vi "CAN MESSAGE WITHOUT START SESSION.vi"(0 "Write":refnum<k21>, 1 "Read":refnum<k21>, 2 "CAN frame":T1 {"payload" format="%x"; "timestamp" format="%<%.7X\n%x>T"; "type" items=["CAN Data"=0, "CAN Remote"=1, "CAN Bus Error"=2, "CAN 2.0 Data"=8, "CAN FD Data"=16, "CAN FD+BRS Data"=24, "J1939 Data"=192, "Delay"=224, "Log Trigger"=225, "Start Trigger"=226]; "identifier" format="%x"}) -> (3 "cluster":T3 {"data[0]"."payload" format="%x"; "data[0]"."timestamp" format="%<%.7X\n%x>T"; "data[0]"."type" items=["CAN Data"=0, "CAN Remote"=1, "CAN Bus Error"=2, "CAN 2.0 Data"=8, "CAN FD Data"=16, "CAN FD+BRS Data"=24, "J1939 Data"=192, "Delay"=224, "Log Trigger"=225, "Start Trigger"=226]; "data[0]"."identifier" format="%x"; "data[1]"."payload" format="%x"; "data[1]"."timestamp" format="%<%.7X\n%x>T"; "data[1]"."type" items=["CAN Data"=0, "CAN Remote"=1, "CAN Bus Error"=2, "CAN 2.0 Data"=8, "CAN FD Data"=16, "CAN FD+BRS Data"=24, "J1939 Data"=192, "Delay"=224, "Log Trigger"=225, "Start Trigger"=226]; "data[1]"."identifier" format="%x"; "data[2]"."payload" format="%x"; "data[2]"."timestamp" format="%<%.7X\n%x>T"; "data[2]"."type" items=["CAN Data"=0, "CAN Remote"=1, "CAN Bus Error"=2, "CAN 2.0 Data"=8, "CAN FD Data"=16, "CAN FD+BRS Data"=24, "J1939 Data"=192, "Delay"=224, "Log Trigger"=225, "Start Trigger"=226]; "data[2]"."identifier" format="%x"; "data[3]"."payload" format="%x"; "data[3]"."timestamp" format="%<%.7X\n%x>T"; "data[3]"."type" items=["CAN Data"=0, "CAN Remote"=1, "CAN Bus Error"=2, "CAN 2.0 Data"=8, "CAN FD Data"=16, "CAN FD+BRS Data"=24, "J1939 Data"=192, "Delay"=224, "Log Trigger"=225, "Start Trigger"=226]; "data[3]"."identifier" format="%x"; "data[4]"."payload" format="%x"; "data[4]"."timestamp" format="%<%.7X\n%x>T"; "data[4]"."type" items=["CAN Data"=0, "CAN Remote"=1, "CAN Bus Error"=2, "CAN 2.0 Data"=8, "CAN FD Data"=16, "CAN FD+BRS Data"=24, "J1939 Data"=192, "Delay"=224, "Log Trigger"=225, "Start Trigger"=226]; "data[4]"."identifier" format="%x"; "data[5]"."payload" format="%x"; "data[5]"."timestamp" format="%<%.7X\n%x>T"; "data[5]"."type" items=["CAN Data"=0, "CAN Remote"=1, "CAN Bus Error"=2, "CAN 2.0 Data"=8, "CAN FD Data"=16, "CAN FD+BRS Data"=24, "J1939 Data"=192, "Delay"=224, "Log Trigger"=225, "Start Trigger"=226]; "data[5]"."identifier" format="%x"; "data[6]"."payload" format="%x"; "data[6]"."timestamp" format="%<%.7X\n%x>T"; "data[6]"."type" items=["CAN Data"=0, "CAN Remote"=1, "CAN Bus Error"=2, "CAN 2.0 Data"=8, "CAN FD Data"=16, "CAN FD+BRS Data"=24, "J1939 Data"=192, "Delay"=224, "Log Trigger"=225, "Start Trigger"=226]; "data[6]"."identifier" format="%x"; "data[7]"."payload" format="%x"; "data[7]"."timestamp" format="%<%.7X\n%x>T"; "data[7]"."type" items=["CAN Data"=0, "CAN Remote"=1, "CAN Bus Error"=2, "CAN 2.0 Data"=8, "CAN FD Data"=16, "CAN FD+BRS Data"=24, "J1939 Data"=192, "Delay"=224, "Log Trigger"=225, "Start Trigger"=226]; "data[7]"."identifier" format="%x"; "data[8]"."payload" format="%x"; "data[8]"."timestamp" format="%<%.7X\n%x>T"; "data[8]"."type" items=["CAN Data"=0, "CAN Remote"=1, "CAN Bus Error"=2, "CAN 2.0 Data"=8, "CAN FD Data"=16, "CAN FD+BRS Data"=24, "J1939 Data"=192, "Delay"=224, "Log Trigger"=225, "Start Trigger"=226]; "data[8]"."identifier" format="%x"}, 4 "Write":refnum<k21>, 5 "Read":refnum<k21>, 6 "error out":errorcluster)   [LabVIEW 2023]
uses:
  <vilib>/xnet/xnet.llb/XNET Frame CAN.ctl
  <vilib>/xnet/xnet.llb/XNET Frame Type CAN.ctl
  <vilib>/xnet/xnet.llb/XNET Write (Frame CAN).vi
  Sub VIs/Global .vi
  <vilib>/xnet/xnet.llb/XNET Read (Frame CAN).vi
panel:
  out "number":u32 format="%x"
  out "data[0].identifier":u32 format="%x"
  in  "error out 2":errorcluster
  out "data 2":T1[](array[typedef]) {"payload" format="%x"; "timestamp" format="%<%.7X\n%x>T"; "type" items=["CAN Data"=0, "CAN Remote"=1, "CAN Bus Error"=2, "CAN 2.0 Data"=8, "CAN FD Data"=16, "CAN FD+BRS Data"=24, "J1939 Data"=192, "Delay"=224, "Log Trigger"=225, "Start Trigger"=226]; "identifier" format="%x"}
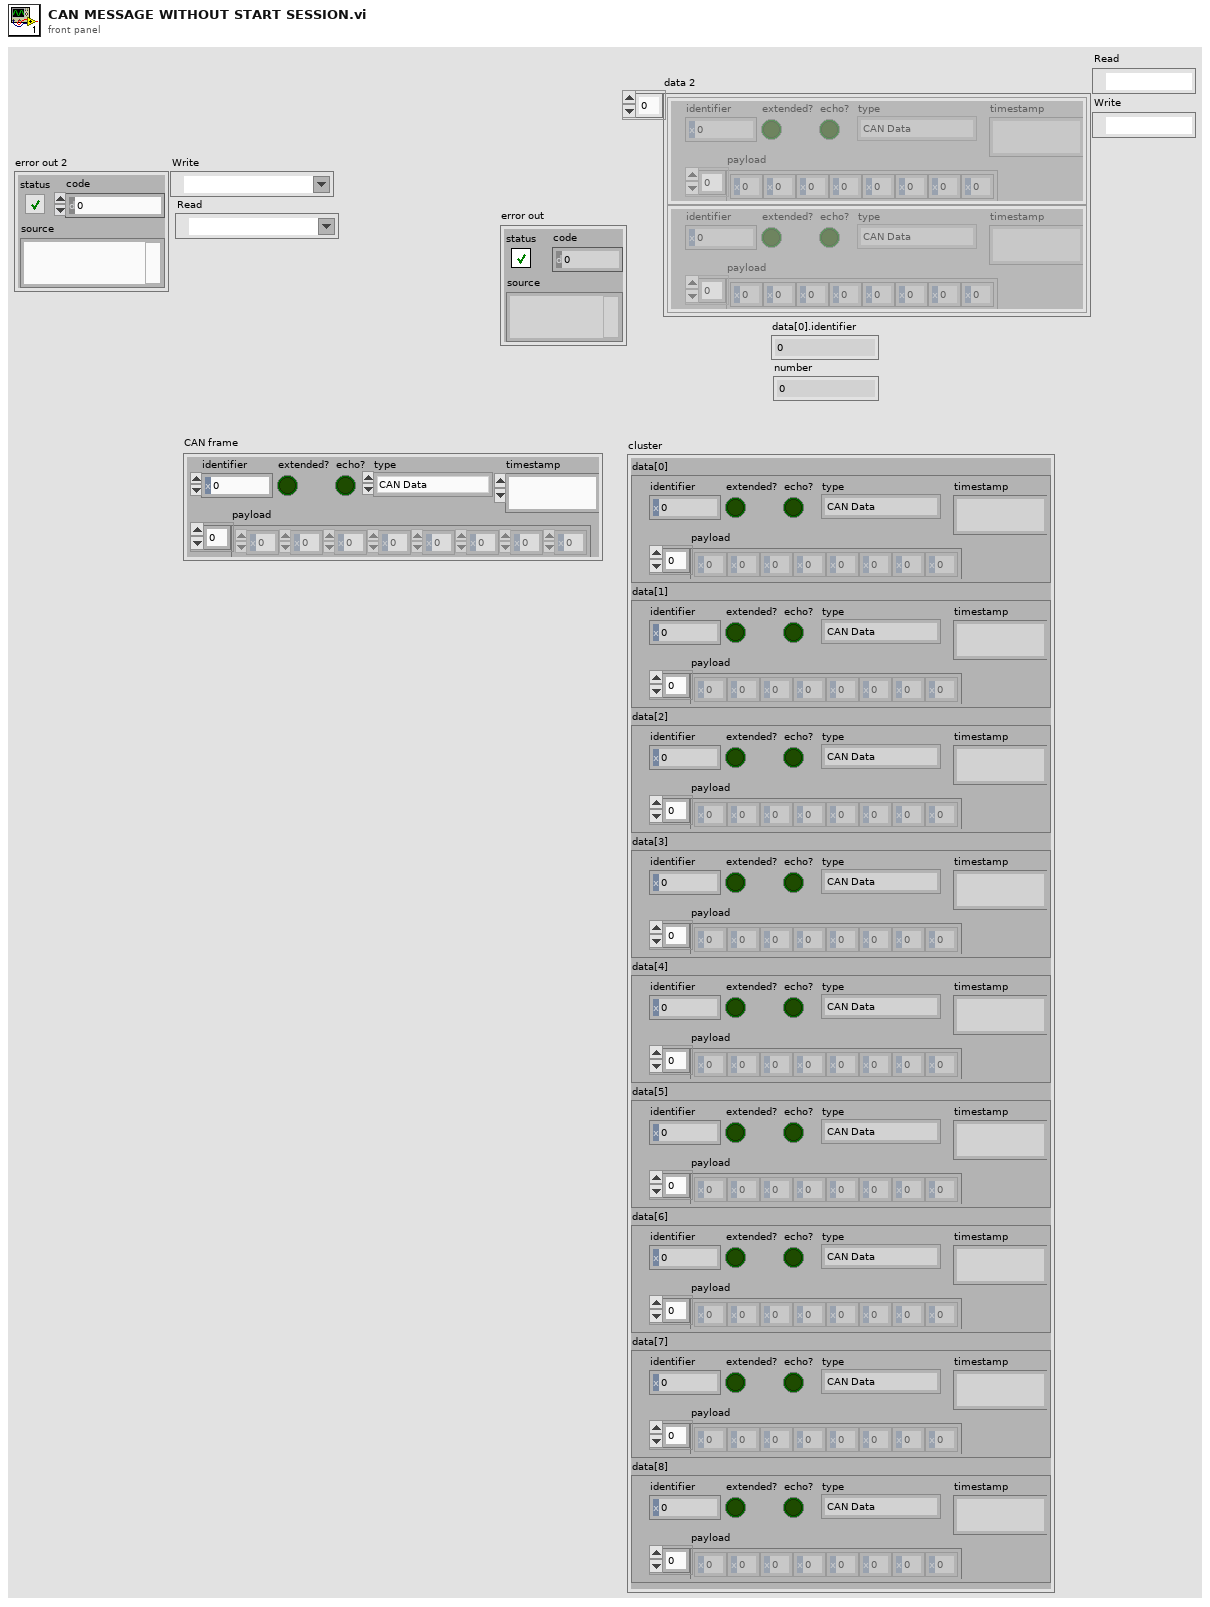
[diagram p1: front panel]
types:
  T1 = typedef "XNET Frame CAN.ctl" = cluster{"timestamp":timestamp, "payload":u8[], "identifier":u32, "type":T2, "extended?":bool, "echo?":bool}
  T2 = typedef "XNET Frame Type CAN.ctl" = u8
  T3 = cluster{"data[0]":T1, "data[1]":T1, "data[2]":T1, "data[3]":T1, "data[4]":T1, "data[5]":T1, "data[6]":T1, "data[7]":T1, "data[8]":T1}
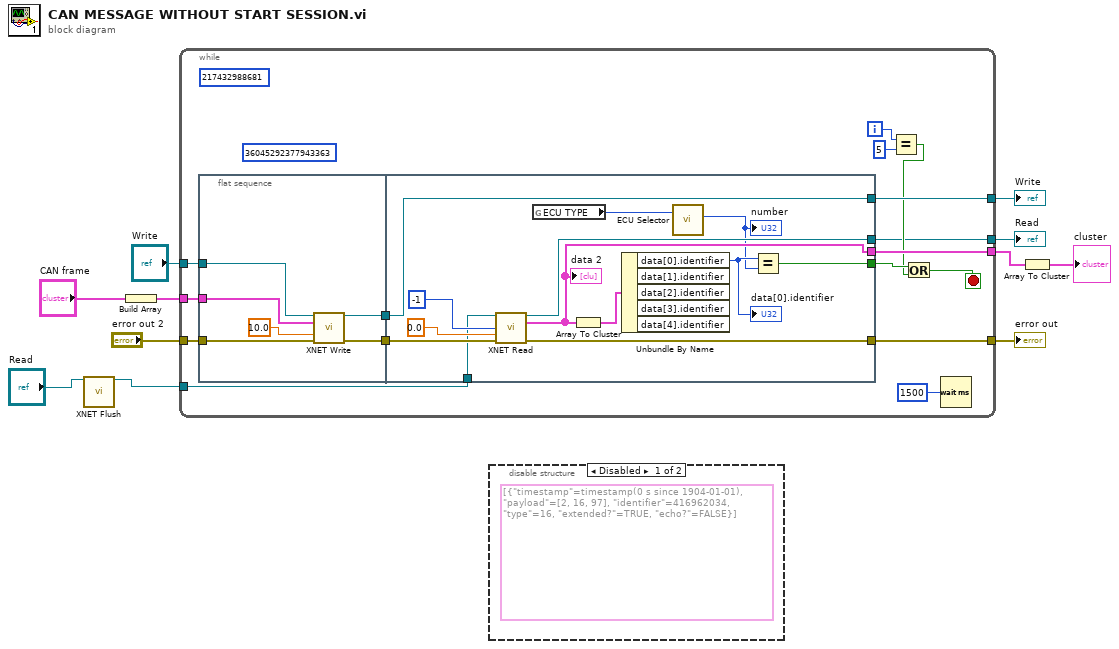
[diagram p0: block diagram]
diagram:
  n1 = call <vilib>:"XNET Flush.vi"("session in"="Read") -> ("session out"=w1:refnum<k21>)  [unwired: 13 in, 1 out]
  n2 = Build Array("CAN frame") -> (w8:T1[])
  n3 = while {
    tunnel: w1 -> [w13]
    tunnel: "Write" -> [w27]
    tunnel: "error out 2" -> [w26]
    tunnel: [w23] -> w7
    tunnel: [w22] -> w11
    tunnel: w8 -> [w21]
    tunnel: [w20] -> w4
    tunnel: [w14] -> w3
    i -> [w17]
    stop <- w12 stop-if-true
    (unwired) u64 36045292377943363 ("Interface:CAN:64bit FD Baud Rate")
    (unwired) u64 217432988681 ("Interface:64bit Baud Rate")
    n4 = flat-sequence {
      tunnel: w27 -> [w33]
      tunnel: w26 -> [w31]
      tunnel: [w30] -> w25
      tunnel: w21 -> [w29]
      tunnel: [w28] -> w19
      tunnel: [w43] -> w18
      tunnel: w25 -> [w42]
      tunnel: w13 -> [w41]
      tunnel: [w40] -> w23
      tunnel: [w39] -> w22
      tunnel: [w37] -> w14
      tunnel: [w36] -> w20
      tunnel: w19 -> [w36]
      frame #0 {
        n5 = call-poly <vilib>:"XNET Write.vi"("session in"=w33, "data"=w29, "timeout (10)"=10.0, "error in (no error)"=w31) -> ("session out"=w28:refnum<k21>, "error out"=w30:errorcluster)  [unwired: 10 in]
      }
      frame #1 {
        n6 = call-poly <vilib>:"XNET Read.vi"("session in"=w41, "number to read (-1)"=-1, "timeout (0)"=0.0, "error in (no error)"=w42) -> ("session out"=w37:refnum<k21>, "data"=w39:T1[], "error out"=w40:errorcluster)  [unwired: 8 in, 1 out]
        "data 2" <- w39
        n7 = global read "Global .vi" "ECU TYPE"() -> (w35:u16)
        n8 = Array To Cluster(array=w39) -> (cluster=w38:T3)
        n9 = Unbundle By Name(w38) -> ("data[0].identifier"=w44:u32)  [unwired: 4 out]
        "data[0].identifier" <- w44
        n10 = call "ECU Selector.vi"("ECU TYPE"=w35) -> ("Numeric Request"=w34:i32)  [unwired: 1 in, 4 out]
        "number" <- w34
        n11 = Equal?(x=w44, y=w34) -> (x = y?=w43:bool)
      }
    }
    n12 = Equal?(x=w17, y=5) -> (x = y?=w16:bool)
    n13 = Or(x=w18, y=w16) -> (x .or. y?=w12:bool)
    n14 = Wait (ms)(milliseconds to wait=u32 1500) -> ()  [unwired: 1 out]
  }
  "error out" <- w7
  "Read" <- w3
  "Write" <- w4
  n15 = disable-structure shown="Disabled" {
    frame Disabled {
      (unwired) T1[] [{"timestamp"=timestamp(0 s since 1904-01-01), "payload"=[2, 16, 97], "identifier"=416962034, "type"=16, "extended?"=TRUE, "echo?"=FALSE}] ("data")
    }
    frame Enabled {
    }
  }
  n16 = Array To Cluster(array=w11) -> (cluster=→"cluster":T3)
